vi "TestM1M3OuterLoopClock.vi"() -> ()   [LabVIEW 2016]
uses:
  <vilib>/FPGAPlugInAG/Dynamic/niLvFpga_Close_Dynamic.vi
  <vilib>/Utility/error.llb/Error Cluster From Error Code.vi
  <vilib>/rvi/errors/niLvFpgaAdjustHostInterfaceError.vi
  <vilib>/RVI Host/nirviSupport.llb/nirviErrorClusterFromErrorCode.vi
  <vilib>/FPGAPlugInAG/Dynamic/niLvFpga_Run_Dynamic.vi
  <vilib>/FPGAPlugInAG/Dynamic/niLvFpga_Reset_Dynamic.vi
  <vilib>/FPGAPlugInAG/Dynamic/niLvFpga_Abort_Dynamic.vi
  <vilib>/rvi/interface/common/dynamic/niFpgaDynamicAddResources.vi
  <vilib>/FPGAPlugInAG/cRIO-9039 (Sync)/niLvFpga_Open_cRIO-9039 (Sync).vi
  <vilib>/rvi/interface/nirviCloseFPGA/nirviCloseFPGA.xnode
  <vilib>/rvi/interface/nirviMethod/nirviMethod.xnode
  <vilib>/rvi/interface/nirviOpenFPGA/nirviOpenFPGA.xnode
  FPGA Bitfiles/M1M3Support.lvbitx
  <vilib>/rvi/interface/nirviMethod/StockFPGA_InlinedMethodWaitForMultipleIRQ.vi
  <vilib>/FPGAPlugInAG/Dynamic/niLvFpga_WaitOnIrq_Dynamic.vi
  <vilib>/FPGAPlugInAG/Dynamic/niLvFpga_AcknowledgeIrq_Dynamic.vi
panel:
  out "Timed Out":bool
  out "LastTime (us)":u32
  in  "Boolean":bool
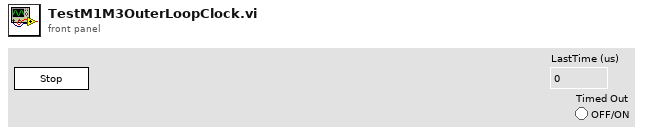
[diagram p1: front panel]
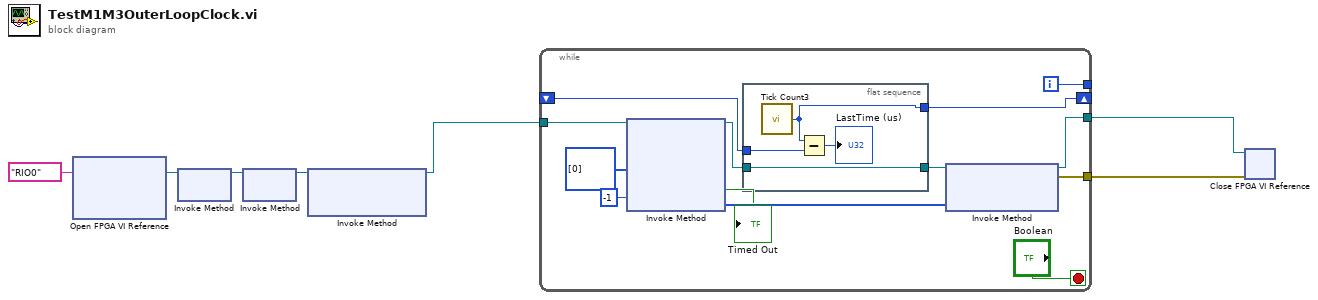
[diagram p0: block diagram]
diagram:
  n1 = xnode "Open FPGA VI Reference"("resource name"=tag "RIO0") -> ("FPGA VI Reference Out"=w7:refnum<k20>)  [unwired: 1 in, 1 out]
  n2 = xnode "Invoke Method"("FPGA VI Reference In"=w7) -> ("FPGA VI Reference Out"=w6:refnum<k20>)  [unwired: 1 in, 1 out]
  n3 = xnode "Invoke Method"("FPGA VI Reference In"=w6) -> ("FPGA VI Reference Out"=w5:refnum<k20>)  [unwired: 1 in, 1 out]
  n4 = xnode "Invoke Method"("FPGA VI Reference In"=w5) -> ("FPGA VI Reference Out"=w4:refnum<k20>)  [unwired: 2 in, 1 out]
  n5 = while {
    tunnel: w4 -> [w14]
    tunnel: [w17] -> w1
    tunnel: [w16] -> w3
    tunnel: [w15] -> _
    shift-right: [w11] -> _
    shift-left: _ -> [w10]
    i -> [w15]
    stop <- "Boolean" stop-if-true
    n6 = xnode "Invoke Method"("FPGA VI Reference In"=w14, "IRQ Number(s)"=i32[] [0], "Timeout (ms)"=-1) -> ("FPGA VI Reference Out"=w12:refnum<k20>, "Timed Out"=→"Timed Out":bool, "IRQ(s) Asserted"=w19:i32[])  [unwired: 1 in, 1 out]
    n7 = flat-sequence {
      tunnel: [w24] -> w13
      tunnel: w12 -> [w24]
      tunnel: [w23] -> w11
      tunnel: w10 -> [w22]
      frame #0 {
        n8 = call "Tick Count3"() -> ("Tick Count(uSec)"=w23:u32)
        n9 = Subtract(x=w23, y=w22) -> (x-y=→"LastTime (us)":u32)
      }
    }
    n10 = xnode "Invoke Method"("FPGA VI Reference In"=w13, "IRQ Number(s)"=w19) -> ("FPGA VI Reference Out"=w16:refnum<k20>, "error out"=w17:errorcluster)  [unwired: 1 in]
  }
  n11 = xnode "Close FPGA VI Reference"("FPGA VI Reference In"=w3, "error in"=w1) -> ()  [unwired: 1 out]
